vi "Save Current Setup File.vi"(8 "error in (no error)":errorcluster, 10 "Setup File":string, 11 "VISA resource name":refnum<visa-resource-name>) -> (0 "error out":errorcluster, 3 "VISA resource name out":refnum<visa-resource-name>)   [LabVIEW 2010, in "Temptronic TP04300.lvlib"]
doc: "This VI saves the current values of the test parameters to the setup file named as in Setup File Name control.\n\nNote: If the file already exists, it will be overwritten.\n\nNote: After sending this command, wait 2 seconds before sending another command."
uses:
  Temptronic TP04300.lvlib
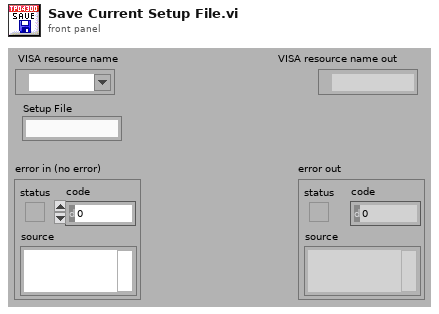
[diagram p1: front panel]
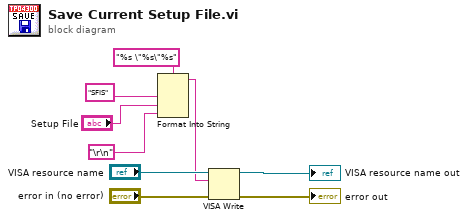
[diagram p0: block diagram]
diagram:
  n1 = Format Into String(format string="%s \"%s\"%s", "SFIS" ("format string"), "Setup File", "\r\n") -> (resulting string=w5:string)  [unwired: 2 in, 1 out]
  n2 = VISA Write(VISA resource name="VISA resource name", write buffer=w5, error in (no error)="error in (no error)") -> (VISA resource name out=→"VISA resource name out":refnum<visa-resource-name>, error out=→"error out":errorcluster)  [unwired: 1 out]
